vi "svx_Polar_Draw_IndicationArcs.vi"(4 "shaft rotating direction":u16, 6 "probe angle [deg]":u16, 8 "grid measurements":T2={"pixel center"={"x"=0, "y"=0}, "scale factors"={"a"=0.0, "b"=0.0, "log?(F)"=FALSE}, "grid color"=16860, "start angle"=0.0, "end angle"=360.0, "tick length"=0, "pixel radius"=0} {"end angle" format="%0.2f"; "start angle" format="%0.2f"; "scale factors"."b" format="%0.2f"; "scale factors"."a" format="%0.2f"}, 9 "Indication Arcs":T1, 10 "width/max":dbl, 11 "Picture":picture) -> (3 "new picture":picture)   [LabVIEW 2017, in "SVX Polar Plot.xctl"]
uses:
  <vilib>/addons/_XControls/Polar Plot/SVX Polar Plot.xctl
  <vilib>/addons/_XControls/Polar Plot/subVIs/svx_Polar_Indication_Arcs.ctl
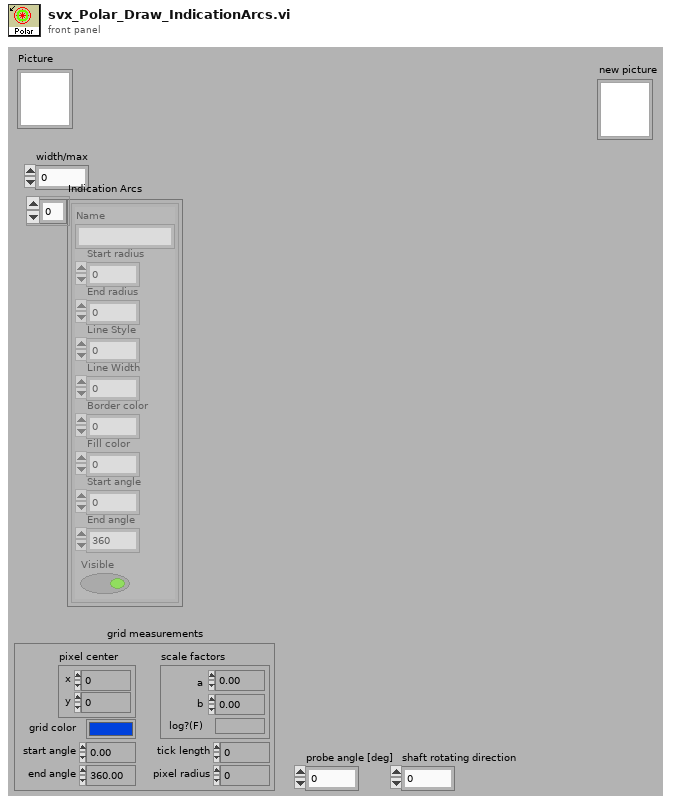
[diagram p1: front panel]
types:
  T1 = typedef "SVX Polar Plot.xctl/svx_Polar_Indication_Arcs.ctl" = cluster{"Name":string, "Start radius":dbl, "End radius":dbl, "Line Style":i32, "Line Width":i32, "Border color":u32, "Fill color":u32, "Start angle":i16, "End angle":i16, "Visible":bool}[]
  T2 = cluster{"pixel center":cluster{"x":i16, "y":i16}, "scale factors":cluster{"a":dbl, "b":dbl, "log?(F)":bool}, "grid color":u32, "start angle":dbl, "end angle":dbl, "tick length":i16, "pixel radius":i32}
  T3 = cluster{"Width":u16, "Style":enum32{"Solid", "Dash", "Dot", "DashDot", "DashDotDot"}}
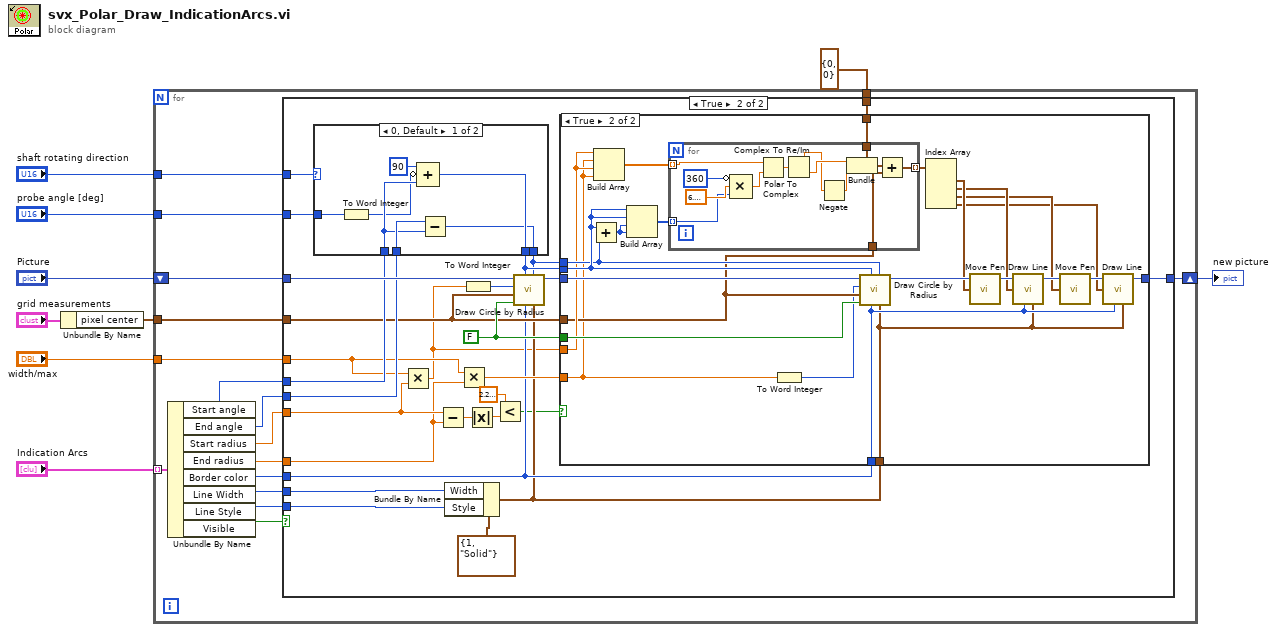
[diagram p0: block diagram]
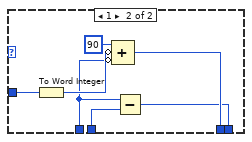
[diagram p4: hidden frame]
diagram:
  n1 = Unbundle By Name("grid measurements") -> ("pixel center"=w6:cluster{"x":i16, "y":i16})
  n2 = for {
    tunnel: "Indication Arcs" -> [w25] mode=indexing
    tunnel: "width/max" -> [w23]
    tunnel: w6 -> [w22]
    shift-right: [w17] -> w5
    shift-left: "Picture" -> [w20]
    tunnel: "shaft rotating direction" -> [w13]
    tunnel: "probe angle [deg]" -> [w14]
    tunnel: cluster{"x":i16, "y":i16} {"x"=0, "y"=0} ("cluster") -> [w10]
    n3 = Unbundle By Name(w25) -> ("Start angle"=w15:i16, "End angle"=w16:i16, "Start radius"=w24:dbl, "End radius"=w11:dbl, "Border color"=w21:u32, "Line Width"=w19:i32, "Line Style"=w18:i32, "Visible"=w12:bool)
    n4 = case shown="True" w12 {
      tunnel: w24 -> [_ w35]
      tunnel: w23 -> [_ w45]
      tunnel: w22 -> [_ w39]
      tunnel: w21 -> [_ w37]
      tunnel: w20 -> [w26 w52]
      tunnel: w19 -> [_ w51]
      tunnel: w18 -> [_ w50]
      tunnel: [w26 w43] -> w17
      tunnel: w16 -> [_ w49]
      tunnel: w15 -> [_ w48]
      tunnel: w14 -> [_ w47]
      tunnel: w13 -> [_ w46]
      tunnel: w11 -> [_ w34]
      tunnel: w10 -> [_ w27]
      frame False {
      }
      frame True {
        w40 = FALSE ("fill?(F)")
        n5 = case shown="0, Default" w46 {
          tunnel: [w97 w104] -> w42
          tunnel: w49 -> [w96 w99]
          tunnel: w48 -> [w95 w100]
          tunnel: [w94 w103] -> w41
          tunnel: w47 -> [w93 w102]
          frame 0, Default {
            n6 = To Word Integer(number=w93) -> (16bit integer=w92:i16)
            n7 = Compound Arithmetic op=ADD(i16 90 ("value"), invert w92, w95) -> (w97:i16)
            n8 = Subtract(x=w96, y=w95) -> (x-y=w94:i16)
          }
          frame 1 {
            n9 = To Word Integer(number=w102) -> (16bit integer=w101:i16)
            n10 = Compound Arithmetic op=ADD(i16 90 ("value"), invert w101, invert w100) -> (w104:i16)
            n11 = Subtract(x=w100, y=w99) -> (x-y=w103:i16)
          }
        }
        n12 = Multiply(x=w45, y=w35) -> (x*y=w29:dbl)
        n13 = Subtract(x=w35, y=w34) -> (x-y=w33:dbl)
        n14 = Bundle By Name(cluster=T3 {"Width"=1, "Style"=enum."Solid"} ("pen"), "Width"=w51, "Style"=w50) -> (w36:T3)
        n15 = Multiply(x=w45, y=w34) -> (x*y=w38:dbl)
        n16 = To Word Integer(number=w29) -> (16bit integer=w28:i16)
        n17 = Absolute Value(x=w33) -> (abs(x)=w32:dbl)
        n18 = Less?(x=2.220446049250313e-16, y=w32) -> (x < y?=w30:bool)
        n19 = call <vilib>:"Draw Circle by Radius.vi"("pen"=w36, "arc size(360)"=w41, "color(black)"=w37, "start angle(0)"=w42, "fill?(F)"=w40, "pixel center"=w39, "radius"=w28, "picture"=w52) -> ("new picture"=w44:picture)  [unwired: 3 in]
        n20 = case shown="True" w30 {
          tunnel: w44 -> [w54 w78]
          tunnel: [w54 w58] -> w43
          tunnel: w42 -> [_ w63]
          tunnel: w41 -> [_ w62]
          tunnel: w40 -> [_ w77]
          tunnel: w39 -> [_ w60]
          tunnel: w38 -> [_ w57]
          tunnel: w37 -> [_ w64]
          tunnel: w36 -> [_ w59]
          tunnel: w29 -> [_ w61]
          tunnel: w27 -> [_ w55]
          frame False {
          }
          frame True {
            n21 = Add(x=w63, y=w62) -> (x+y=w74:i16)
            n22 = Build Array(w61, w57, w61, w57) -> (w72:dbl[])
            n23 = Build Array(w63, w63, w74, w74) -> (w73:i16[])
            n24 = for {
              tunnel: w60 -> [w86]
              tunnel: w73 -> [w85] mode=indexing
              tunnel: w72 -> [w84] mode=indexing
              tunnel: [w83] -> w71 mode=indexing
              tunnel: w55 -> [w79]
              n25 = Compound Arithmetic op=MULTIPLY(invert i16 360 ("value"), 6.283185307179586, w85) -> (w89:dbl)
              n26 = Polar To Complex(1:w89, 2:w84) -> (0:w88:cdb)
              n27 = Complex To Re/Im(x + iy=w88) -> (x=w81:dbl, y=w82:dbl)
              n28 = Negate(x=w81) -> (-x=w80:dbl)
              n29 = Bundle(cluster=w79, "x"=w82, "y"=w80) -> (w87:cluster{"x":i16, "y":i16})
              n30 = Add(x=w87, y=w86) -> (x+y=w83:cluster{"x":i16, "y":i16})
            }
            n31 = To Word Integer(number=w57) -> (16bit integer=w56:i16)
            n32 = call <vilib>:"Draw Circle by Radius.vi"("pen"=w59, "arc size(360)"=w62, "color(black)"=w64, "start angle(0)"=w63, "fill?(F)"=w77, "pixel center"=w60, "radius"=w56, "picture"=w78) -> ("new picture"=w76:picture)  [unwired: 3 in]
            n33 = Index Array(array=w71) -> (element #1=w70:cluster{"x":i16, "y":i16}, element #2=w69:cluster{"x":i16, "y":i16}, element #3=w66:cluster{"x":i16, "y":i16}, element #4=w65:cluster{"x":i16, "y":i16})  [unwired: 4 in]
            n34 = call <vilib>:"Move Pen.vi"("new position"=w70, "picture"=w76) -> ("new picture"=w75:picture)  [unwired: 3 in]
            n35 = call <vilib>:"Draw Line.vi"("picture"=w75, "end point"=w69, "color(black)"=w64, "pen"=w59) -> ("new picture"=w67:picture)  [unwired: 5 in]
            n36 = call <vilib>:"Move Pen.vi"("new position"=w66, "picture"=w67) -> ("new picture"=w68:picture)  [unwired: 3 in]
            n37 = call <vilib>:"Draw Line.vi"("picture"=w68, "end point"=w65, "color(black)"=w64, "pen"=w59) -> ("new picture"=w58:picture)  [unwired: 5 in]
          }
        }
      }
    }
  }
  "new picture" <- w5
